vi "Config Integration.vi"(0 "VISA resource name":refnum<visa-resource-name>, 1 "Integ Type (0: Standard)":u16(ring) items=["Standard", "Advanced"], 5 "Integ Mode (0: Normal)":u16(ring) items=["Normal", "Continuous"], 7 "Hour (0)":u32 max=10000, 9 "Minute (0)":u32 max=59 step=1, 11 "error in (no error)":errorcluster, 12 "Second (0)":u32 max=59 step=1) -> (4 "VISA resource name out":refnum<visa-resource-name>, 15 "error out":errorcluster)   [LabVIEW 2013, in "Yokogawa WT200 Series.lvlib"]
doc: "This VI sends the Integration command to the WT200 Series."
uses:
  <instrlib>/Yokogawa WT200 Series/Yokogawa WT200 Series.lvlib
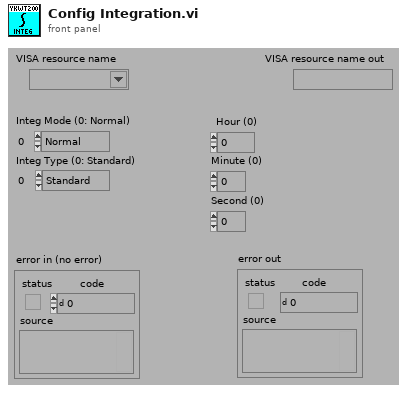
[diagram p1: front panel]
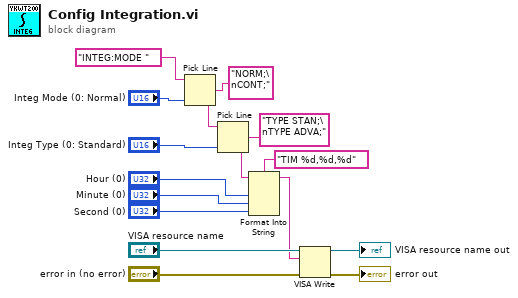
[diagram p0: block diagram]
diagram:
  n1 = Pick Line(string ("")="INTEG:MODE ", multi-line string="NORM;\nCONT;", line index="Integ Mode (0: Normal)") -> (output string=w4:string)
  n2 = Pick Line(string ("")=w4, multi-line string="TYPE STAN;\nTYPE ADVA;", line index="Integ Type (0: Standard)") -> (output string=w3:string)
  n3 = Format Into String(format string="TIM %d,%d,%d", initial string=w3, "Hour (0)", "Minute (0)", "Second (0)") -> (resulting string=w7:string)  [unwired: 1 in, 1 out]
  n4 = VISA Write(VISA resource name="VISA resource name", write buffer=w7, error in (no error)="error in (no error)") -> (VISA resource name out=→"VISA resource name out":refnum<visa-resource-name>, error out=→"error out":errorcluster)  [unwired: 1 out]
